vi "readfromexel.vi"(8 "RANGE":string="A10:H18", 9 "Path":path) -> (3 "Element 1":string[][](array[string]))   [LabVIEW 2012]
panel:
  in  "Excel._Worksheet 2":refnum<k7>
  in  "Excel._Application":refnum<k7>
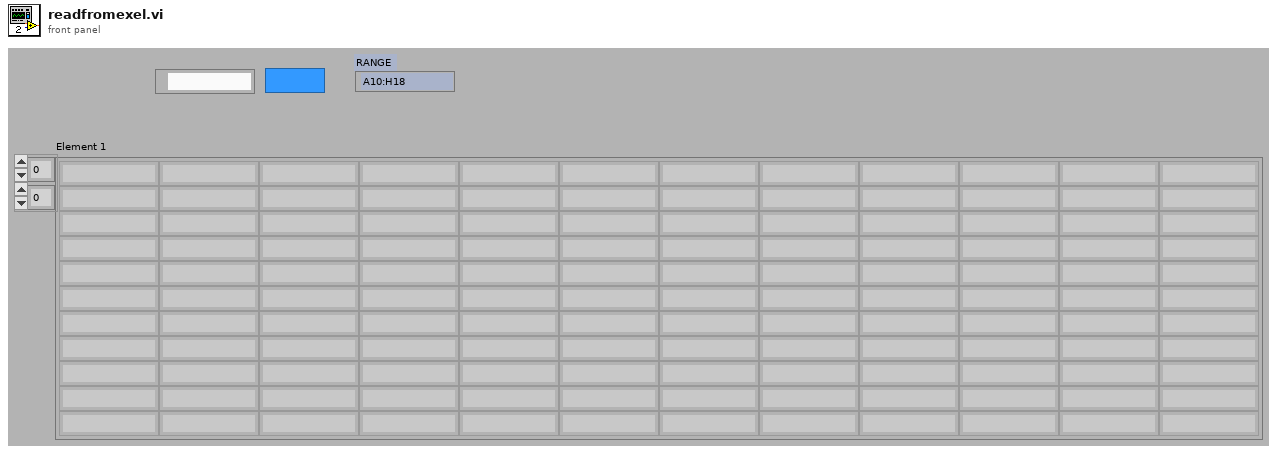
[diagram p1: front panel]
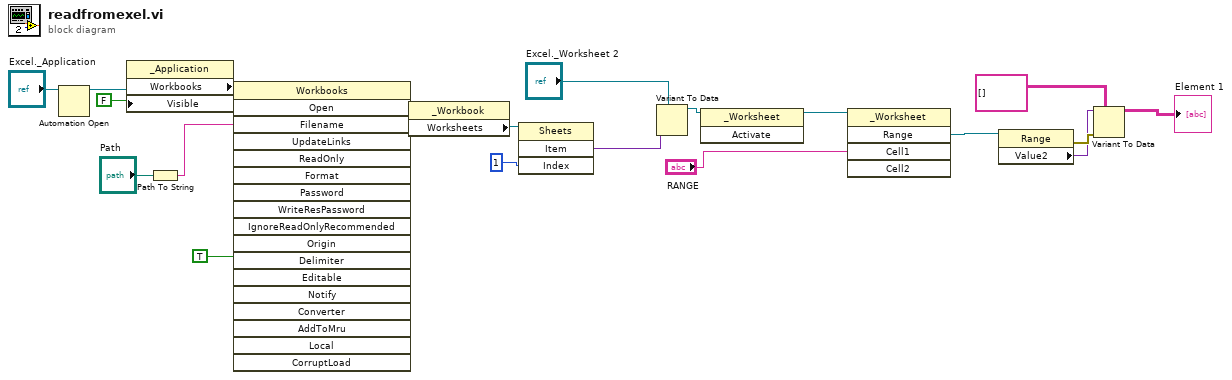
[diagram p0: block diagram]
diagram:
  n1 = Automation Open(Automation Refnum="Excel._Application") -> (Automation Refnum=w20:refnum<k7>)  [unwired: 3 in, 1 out]
  n2 = property class="_Application"(reference=w20, "Visible"=FALSE) -> ("Workbooks"=w18:refnum<k7>)  [unwired: 1 in, 2 out]
  n3 = Path To String(path="Path") -> (string=w17:string)
  n4 = invoke class="Workbooks" method="Open"(reference=w18, "Filename"=w17, "Editable"=TRUE) -> ("Open"=w11:refnum<k7>)  [unwired: 15 in, 17 out]
  n5 = property class="_Workbook"(reference=w11) -> ("Worksheets"=w10:refnum<k7>)  [unwired: 1 in, 2 out]
  n6 = invoke class="Sheets" method="Item"(reference=w10, "Index"=1) -> ("Item"=w13:variant)  [unwired: 2 in, 3 out]
  n7 = Variant To Data(type="Excel._Worksheet 2", Variant=w13) -> (data=w16:refnum<k7>)  [unwired: 1 in, 1 out]
  n8 = invoke class="_Worksheet" method="Activate"(reference=w16) -> (reference out=w1:refnum<k7>)  [unwired: 2 in, 2 out]
  n9 = invoke class="_Worksheet" method="Range"(reference=w1, "Cell1"="RANGE") -> ("Range"=w3:refnum<k7>)  [unwired: 3 in, 4 out]
  n10 = property class="Range"(reference=w3) -> (error out=w6:errorcluster, "Value2"=w5:variant)  [unwired: 1 in, 1 out]
  n11 = Variant To Data(error in=w6, type=string[][] [] ("Array"), Variant=w5) -> (data=→"Element 1":string[][])  [unwired: 1 out]
